vi "CoboltLaser_LaserOff.vi"(0 "ComPort":refnum<visa-resource-name>, 3 "CheckResponse":bool=TRUE, 7 "error in (no error)":errorcluster) -> (20 "ComPortOut":refnum<visa-resource-name>, 27 "error out":errorcluster)   [LabVIEW 2012, in "Cobolt.lvclass"]
doc: "Use this template to build a VI to use as a subVI."
uses:
  Template/Cobolt.lvclass
panel:
  out "ResponseOK":bool
  out "Response":string
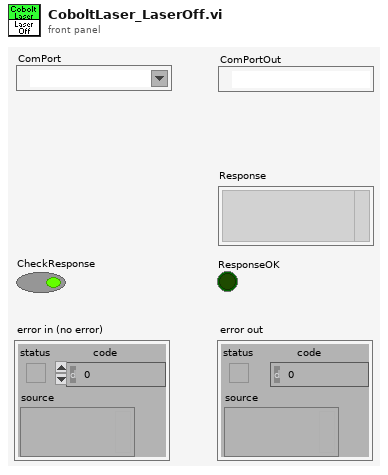
[diagram p1: front panel]
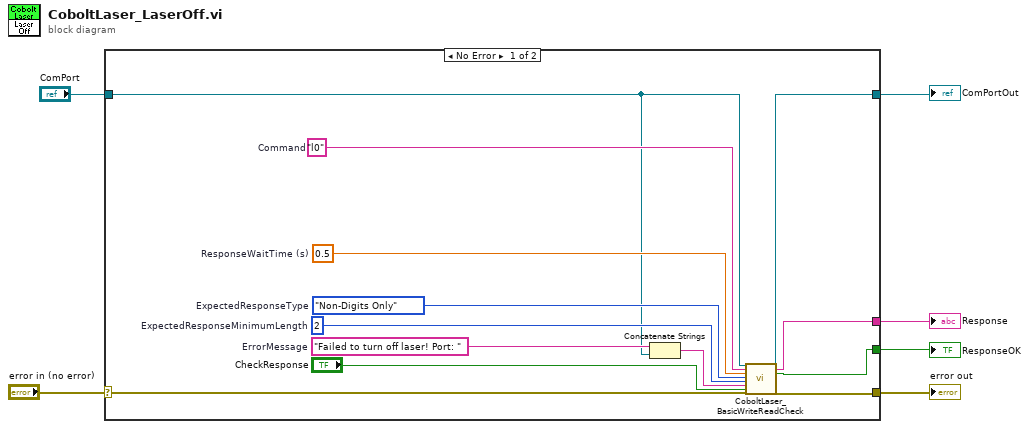
[diagram p0: block diagram]
diagram:
  n1 = case shown="No Error" "error in (no error)" {
    selector: "error in (no error)" -> [w19 w21]
    tunnel: [w18 w21] -> w5
    tunnel: "ComPort" -> [w10 w20]
    tunnel: [w9 w20] -> w3
    tunnel: [w8 _] -> w2
    tunnel: [w7 _] -> w1
    frame No Error {
      w15 = 2  # ExpectedResponseMinimumLength
      w16 = enum16{"Any", "Digits Only", "Non-Digits Only"}."Non-Digits Only"  # ExpectedResponseType
      w17 = 0.5  # ResponseWaitTime (s)
      w13 = "Failed to turn off laser! Port: "  # ErrorMessage
      w11 = "l0"  # Command
      n2 = Concatenate Strings(w13, w10) -> (w12:string)
      n3 = call "CoboltLaser_BasicWriteReadCheck.vi"("ComPort"=w10, "Command"=w11, "ResponseWaitTime (s)"=w17, "ExpectedResponseType"=w16, "ExpectedResponseMinimumLength"=w15, "ErrorMessage"=w12, "CheckResponse"="CheckResponse", "error in (no error)"=w19) -> ("ComPortOut"=w9:refnum<visa-resource-name>, "Response"=w8:string, "ResponseOK"=w7:bool, "error out"=w18:errorcluster)  [unwired: 16 in]
    }
    frame Error {
    }
  }
  "error out" <- w5
  "Response" <- w2
  "ComPortOut" <- w3
  "ResponseOK" <- w1
